vi "DelayLineVI.vi"(8 "error in (no error)":errorcluster, 9 "ControlQueue":refnum<queue>, 11 "DelayLine.lvclass":refnum<class "DelayLine.lvclass">) -> (0 "error out":errorcluster)   [LabVIEW 2019, in "DelayLine.lvclass"]
uses:
  DelayLine.lvclass
  C:/Users/elysium/Documents/dev/TRANCON/Classes/GeneralFunctionality/GeneralFunctionality.lvclass
  dependecies/ControlsVIs/Clusters-def/Message types.ctl
  GeneralFunctionality/GeneralFunctionality.lvclass/GeneralFunctionality.ctl
  Message/Message.lvclass/Message.ctl
  dependecies/ControlsVIs/Clusters-def/Standard Command.ctl
  dependecies/ControlsVIs/Clusters-def/DL-Com-MoveAxis.ctl
  dependecies/ControlsVIs/Clusters-def/SERVER-Commands.ctl
  Message/Message.lvclass
  Control/Control-Server/Control-Server.lvclass
  GeneralFunctionality/GeneralFunctionality.lvclass
panel:
  in  "axisIInum":dbl min=0.0 max=0.0 step=4.0
  in  "axisInum":dbl min=-70.0 max=70.0
  out "Received command":string
  in  "Set Zero":bool
  in  "AxisII":dbl(slide) min=0.0 max=0.0
  in  "AxisI":dbl(slide) min=-70.0 max=70.0 scale=-70.0..70.0
  # "moves in 4mm steps"
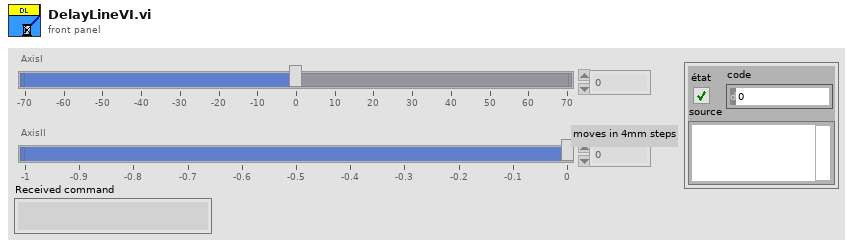
[diagram p1: front panel]
types:
  T1 = typedef "Message types.ctl" = string
  T2 = typedef "Standard Command.ctl" = cluster{"command":string, "data":variant}
  T3 = typedef "DelayLine.lvclass/DL-Com-MoveAxis.ctl" = cluster{"Axis":i32, "Where":dbl, "How":u16}
  T4 = typedef "Control-Server.lvclass/SERVER-Commands.ctl" = string
  T5 = typedef "eventsource.ctl" = u32
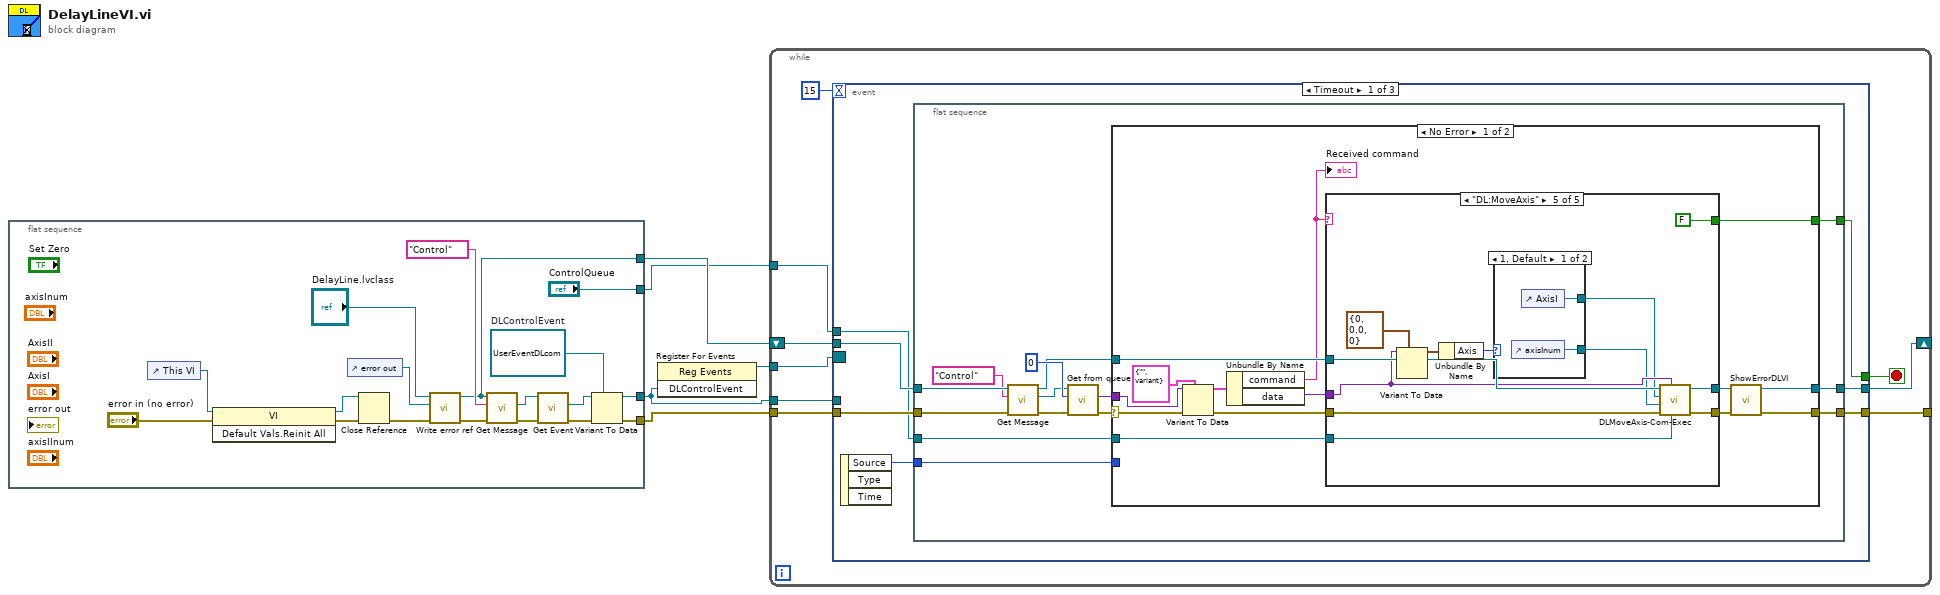
[diagram p0: block diagram]
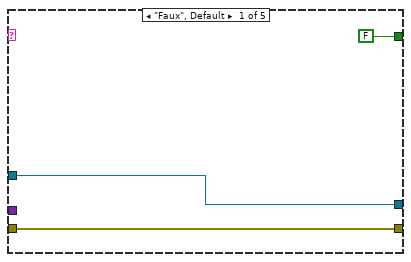
[diagram p2: hidden frame]
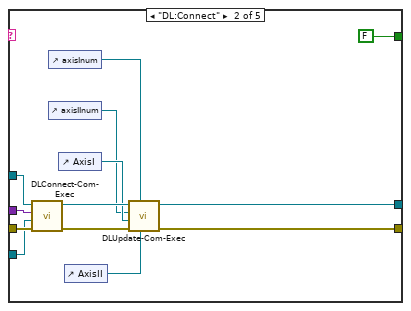
[diagram p3: hidden frame]
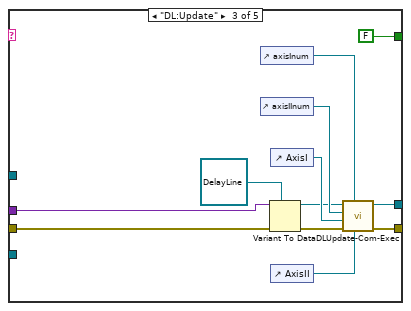
[diagram p4: hidden frame]
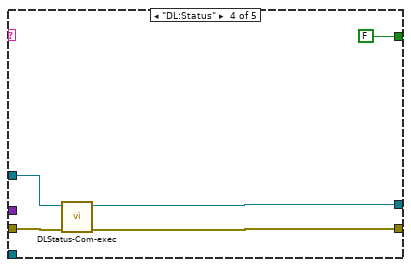
[diagram p5: hidden frame]
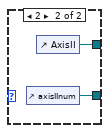
[diagram p6: hidden frame]
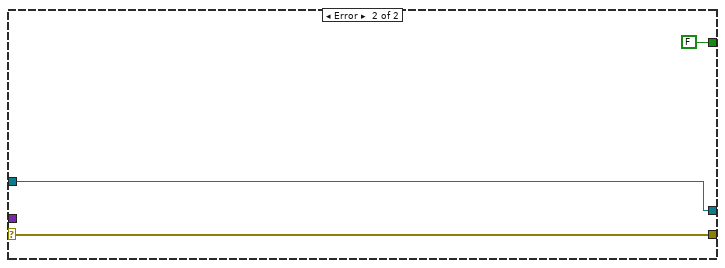
[diagram p7: hidden frame]
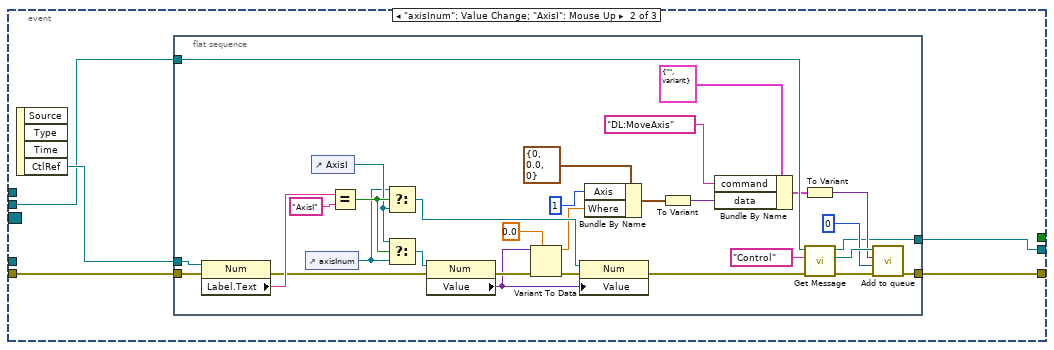
[diagram p8: hidden frame]
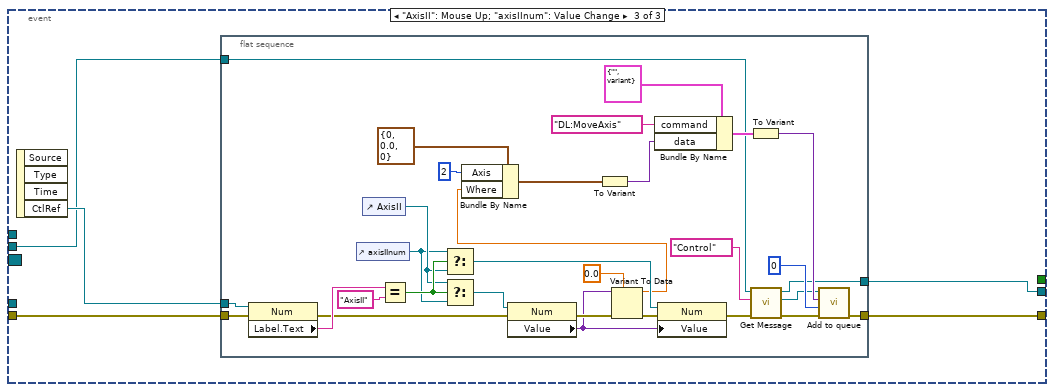
[diagram p9: hidden frame]
diagram:
  n1 = flat-sequence {
    tunnel: [w9] -> w4
    tunnel: ["ControlQueue"] -> w3
    tunnel: [w13] -> w2
    tunnel: [w11] -> w1
    frame #0 {
      w15 = refnum<user-event> refnum  # DLControlEvent
      n2 = control-ref of="This VI"() -> (w21:refnum<vi>)
      n3 = invoke class="VI" method="Default Vals.Reinit All"(reference=w21, error in="error in (no error)") -> (reference out=w22:refnum<vi>, error out=w23:errorcluster)  [unwired: 1 in, 1 out]
      n4 = control-ref of="error out"() -> (w8:refnum<vi>)
      n5 = Close Reference(reference=w22, error in (no error)=w23) -> (error out=w7:errorcluster)
      n6 = call "Write error ref.vi"("error in (no error)"=w7, "error"=w8, "GeneralFunctionality in"="DelayLine.lvclass") -> ("error out"=w6:errorcluster, "GeneralFunctionality out"=w9:refnum<class "DelayLine.lvclass">)  [unwired: 7 in]
      n7 = call "Get Message.vi"("error in (no error)"=w6, "Message type"=T1 "Control", "GeneralFunctionality en entrée"=w9) -> ("error out"=w17:errorcluster, "Message.lvclass"=w19:refnum<class "Message.lvclass">)  [unwired: 6 in, 1 out]
      n8 = call "Get Event.vi"("error in (no error)"=w17, "Message en entrée"=w19) -> ("error out"=w14:errorcluster, "UserEventCommand"=w12:refnum<user-event>)  [unwired: 7 in, 1 out]
      n9 = Variant To Data(error in=w14, type=w15, Variant=w12) -> (data=w11:refnum<user-event>, error out=w13:errorcluster)
    }
  }
  n10 = register-events(w1) -> (reference out=w5:refnum<event-registration>)  [unwired: 2 in, 1 out]
  n11 = while {
    tunnel: w5 -> [w32]
    shift-right: [w31] -> _
    shift-left: w4 -> [w30]
    tunnel: w2 -> [w29]
    tunnel: [w28] -> _
    tunnel: w3 -> [w27]
    tunnel: w1 -> [w25]
    stop <- w24 stop-if-true
    n12 = event shown="[0] Timeout" {
      selector: w32 -> [_ _ _]
      dyn-events: _ -> [_ _ _]
      timeout: 15 -> [_ _ _]
      tunnel: [w37 w121 w157] -> w31
      tunnel: w30 -> [w39 w122 w158]
      tunnel: w29 -> [w38 w123 w159]
      tunnel: [w36 w120 w156] -> w28
      tunnel: w27 -> [w35 _ _]
      tunnel: w25 -> [_ _ _]
      tunnel: [w34 _ _] -> w24
      event Timeout {
        n13 = event-data() -> ("Source"=w33:T5)  [unwired: 1 in, 2 out]
        n14 = flat-sequence {
          tunnel: w39 -> [w53]
          tunnel: w38 -> [w52]
          tunnel: [w45] -> w37
          tunnel: [w44] -> w36
          tunnel: w35 -> [w43]
          tunnel: [w42] -> w34
          tunnel: w33 -> [w40]
          frame #0 {
            n15 = call "Get Message.vi"("error in (no error)"=w52, "Message type"=T1 "Control", "GeneralFunctionality en entrée"=w53) -> ("error out"=w50:errorcluster, "Message.lvclass"=w41:refnum<class "Message.lvclass">, "GeneralFunctionality en sortie"=w46:refnum<class "DelayLine.lvclass">)  [unwired: 6 in]
            n16 = call "Get from queue.vi"("error in (no error)"=w50, "timeout in ms (-1)"=0, "Message in"=w41) -> ("error out"=w47:errorcluster, "Data"=w48:variant)  [unwired: 5 in, 2 out]
            n17 = case shown="No Error" w47 {
              selector: w47 -> [w67 w119]
              tunnel: w48 -> [w59 _]
              tunnel: [w54 w119] -> w44
              tunnel: w46 -> [w62 w118]
              tunnel: [w56 w118] -> w45
              tunnel: w43 -> [w61 _]
              tunnel: [w58 FALSE] -> w42
              tunnel: w40 -> [_ _]
              frame No Error {
                n18 = Variant To Data(error in=w67, type=T2 {"command"="", "data"=variant} ("input cluster"), Variant=w59) -> (data=w65:T2, error out=w63:errorcluster)
                n19 = Unbundle By Name(w65) -> ("command"=w60:string, "data"=w64:variant)
                "Received command" <- w60
                n20 = case shown="\"DL:MoveAxis\"" w60 {
                  tunnel: [w70 w76 w92 w96 w112] -> w57
                  tunnel: [w69 w75 w91 w97 w111] -> w55
                  tunnel: [FALSE FALSE FALSE FALSE FALSE] -> w58
                  tunnel: w64 -> [_ w79 w89 _ w106]
                  tunnel: w63 -> [w69 w82 w87 w98 w110]
                  tunnel: w62 -> [w70 w81 _ w99 w109]
                  tunnel: w61 -> [_ w80 _ _ w101]
                  frame "Faux", Default {
                  }
                  frame "DL:Connect" {
                    n21 = call "DLConnect-Com-Exec.vi"("error in (no error)"=w82, "ControlQueue"=w80, "data"=w79, "DelayLine in"=w81) -> ("error out"=w77:errorcluster, "DelayLine out"=w78:refnum<class "DelayLine.lvclass">)  [unwired: 6 in]
                    n22 = control-ref of="axisInum"() -> (w71:refnum<vi>)
                    n23 = control-ref of="axisIInum"() -> (w72:refnum<vi>)
                    n24 = control-ref of="AxisI"() -> (w73:refnum<vi>)
                    n25 = control-ref of="AxisII"() -> (w74:refnum<vi>)
                    n26 = call "DLUpdate-Com-Exec.vi"("AxisII"=w74, "axisInum"=w71, "error in (no error)"=w77, "AxisI"=w73, "axisIInum"=w72, "DelayLine.lvclass"=w78) -> ("error out"=w75:errorcluster, "DelayLine out"=w76:refnum<class "DelayLine.lvclass">)  [unwired: 4 in]
                  }
                  frame "DL:Update" {
                    n27 = control-ref of="axisInum"() -> (w84:refnum<vi>)
                    n28 = control-ref of="axisIInum"() -> (w94:refnum<vi>)
                    n29 = Variant To Data(error in=w87, type=refnum<class "DelayLine.lvclass"> refnum ("DelayLine out"), Variant=w89) -> (data=w85:refnum<class "DelayLine.lvclass">, error out=w86:errorcluster)
                    n30 = control-ref of="AxisI"() -> (w93:refnum<vi>)
                    n31 = control-ref of="AxisII"() -> (w95:refnum<vi>)
                    n32 = call "DLUpdate-Com-Exec.vi"("AxisII"=w95, "axisInum"=w84, "error in (no error)"=w86, "AxisI"=w93, "axisIInum"=w94, "DelayLine.lvclass"=w85) -> ("error out"=w91:errorcluster, "DelayLine out"=w92:refnum<class "DelayLine.lvclass">)  [unwired: 4 in]
                  }
                  frame "DL:Status" {
                    n33 = call "DLStatus-Com-exec.vi"("error in (no error)"=w98, "DelayLine in"=w99) -> ("error out"=w97:errorcluster, "DelayLine out"=w96:refnum<class "DelayLine.lvclass">)  [unwired: 8 in]
                  }
                  frame "DL:MoveAxis" {
                    n34 = Variant To Data(type=T3 {"Axis"=0, "Where"=0.0, "How"=0} ("output cluster"), Variant=w106) -> (data=w105:T3)  [unwired: 1 in, 1 out]
                    n35 = Unbundle By Name(w105) -> ("Axis"=w104:i32)
                    n36 = case shown="1, Default" w104 {
                      tunnel: [w114 w116] -> w103
                      tunnel: [w113 w115] -> w102
                      frame 1, Default {
                        n37 = control-ref of="axisInum"() -> (w113:refnum<vi>)
                        n38 = control-ref of="AxisI"() -> (w114:refnum<vi>)
                      }
                      frame 2 {
                        n39 = control-ref of="axisIInum"() -> (w115:refnum<vi>)
                        n40 = control-ref of="AxisII"() -> (w116:refnum<vi>)
                      }
                    }
                    n41 = call "DLMoveAxis-Com-Exec.vi"("ControlQueue"=w101, "data"=w106, "error in (no error)"=w110, "axisInum"=w102, "AxisI"=w103, "DelayLine in"=w109) -> ("error out"=w111:errorcluster, "DelayLine out"=w112:refnum<class "DelayLine.lvclass">)  [unwired: 4 in]
                  }
                }
                n42 = call "ShowErrorDLVI.vi"("error in (no error)"=w55, "DelayLine in"=w57) -> ("error out"=w54:errorcluster, "DelayLine out"=w56:refnum<class "DelayLine.lvclass">)  [unwired: 8 in]
              }
              frame Error {
              }
            }
          }
        }
      }
      event "axisInum": Value Change; "AxisI": Mouse Up {
        n43 = event-data() -> ("CtlRef"=w124:refnum<vi>)  [unwired: 1 in, 3 out]
        n44 = flat-sequence {
          tunnel: w124 -> [w155]
          tunnel: w123 -> [w154]
          tunnel: w122 -> [w141]
          tunnel: [w126] -> w121
          tunnel: [w125] -> w120
          frame #0 {
            n45 = property class="Num"(reference=w155, error in=w154) -> (error out=w151:errorcluster, "Label.Text"=w153:string)  [unwired: 1 out]
            n46 = control-ref of="axisInum"() -> (w142:refnum<vi>)
            n47 = control-ref of="AxisI"() -> (w143:refnum<vi>)
            n48 = Equal?(x=w153, y="AxisI") -> (x = y?=w148:bool)
            n49 = Select(t=w142, s=w148, f=w143) -> (s? t:f=w147:refnum<vi>)
            n50 = Select(t=w143, s=w148, f=w142) -> (s? t:f=w150:refnum<vi>)
            n51 = property class="Num"(reference=w150, error in=w151) -> (error out=w149:errorcluster, "Value"=w146:variant)  [unwired: 1 out]
            n52 = Variant To Data(error in=w149, type=0.0, Variant=w146) -> (data=w129:dbl, error out=w145:errorcluster)
            n53 = property class="Num"(reference=w147, error in=w145, "Value"=w146) -> (error out=w140:errorcluster)  [unwired: 1 out]
            n54 = Bundle By Name(cluster=T3 {"Axis"=0, "Where"=0.0, "How"=0} ("output cluster"), "Axis"=1, "Where"=w129) -> (w127:T3)
            n55 = To Variant(anything=w127) -> (Variant=w128:variant)
            n56 = Bundle By Name(cluster=T2 {"command"="", "data"=variant} ("input cluster"), "command"=T4 "DL:MoveAxis" ("Commands"), "data"=w128) -> (w134:T2)
            n57 = To Variant(anything=w134) -> (Variant=w133:variant)
            n58 = call "Get Message.vi"("error in (no error)"=w140, "Message type"=T1 "Control", "GeneralFunctionality en entrée"=w141) -> ("error out"=w138:errorcluster, "Message.lvclass"=w137:refnum<class "Message.lvclass">, "GeneralFunctionality en sortie"=w126:refnum<class "DelayLine.lvclass">)  [unwired: 6 in]
            n59 = call "Add to queue.vi"("error in (no error)"=w138, "timeout in ms (-1)"=0, "Data"=w133, "Message in"=w137) -> ("error out"=w125:errorcluster)  [unwired: 6 in, 1 out]
          }
        }
      }
      event "AxisII": Mouse Up; "axisIInum": Value Change {
        n60 = event-data() -> ("CtlRef"=w160:refnum<vi>)  [unwired: 1 in, 3 out]
        n61 = flat-sequence {
          tunnel: w160 -> [w182]
          tunnel: w159 -> [w181]
          tunnel: w158 -> [w164]
          tunnel: [w163] -> w157
          tunnel: [w162] -> w156
          frame #0 {
            n62 = property class="Num"(reference=w182, error in=w181) -> (error out=w189:errorcluster, "Label.Text"=w191:string)  [unwired: 1 out]
            n63 = control-ref of="axisIInum"() -> (w178:refnum<vi>)
            n64 = control-ref of="AxisII"() -> (w179:refnum<vi>)
            n65 = Equal?(x=w191, y="AxisII") -> (x = y?=w186:bool)
            n66 = Select(t=w178, s=w186, f=w179) -> (s? t:f=w185:refnum<vi>)
            n67 = Select(t=w179, s=w186, f=w178) -> (s? t:f=w188:refnum<vi>)
            n68 = property class="Num"(reference=w188, error in=w189) -> (error out=w187:errorcluster, "Value"=w184:variant)  [unwired: 1 out]
            n69 = Variant To Data(error in=w187, type=0.0, Variant=w184) -> (data=w161:dbl, error out=w183:errorcluster)
            n70 = Bundle By Name(cluster=T3 {"Axis"=0, "Where"=0.0, "How"=0} ("output cluster"), "Axis"=2, "Where"=w161) -> (w177:T3)
            n71 = To Variant(anything=w177) -> (Variant=w176:variant)
            n72 = Bundle By Name(cluster=T2 {"command"="", "data"=variant} ("input cluster"), "command"=T4 "DL:MoveAxis" ("Commands"), "data"=w176) -> (w171:T2)
            n73 = property class="Num"(reference=w185, error in=w183, "Value"=w184) -> (error out=w165:errorcluster)  [unwired: 1 out]
            n74 = To Variant(anything=w171) -> (Variant=w172:variant)
            n75 = call "Get Message.vi"("error in (no error)"=w165, "Message type"=T1 "Control", "GeneralFunctionality en entrée"=w164) -> ("error out"=w167:errorcluster, "Message.lvclass"=w168:refnum<class "Message.lvclass">, "GeneralFunctionality en sortie"=w163:refnum<class "DelayLine.lvclass">)  [unwired: 6 in]
            n76 = call "Add to queue.vi"("error in (no error)"=w167, "timeout in ms (-1)"=0, "Data"=w172, "Message in"=w168) -> ("error out"=w162:errorcluster)  [unwired: 6 in, 1 out]
          }
        }
      }
    }
  }
